vi "add_vi.vi"(8 "error in (no error)":errorcluster, 9 "Path":path, 10 "vi_name":string, 11 "VIGraph in":refnum<class "HierarchyGraph.lvclass">) -> (0 "error out":errorcluster, 1 "VINode out":refnum<class "HierarchyNode.lvclass">, 2 "node already included?":bool, 3 "VIGraph out":refnum<class "HierarchyGraph.lvclass">)   [LabVIEW 2020, in "vi-hierarchy.lvlib" / "HierarchyGraph.lvclass"]
uses:
  HierarchyGraph.lvclass
  C:/Projects/labview-project-load-tools/source/submodules/graph-api-labview/source/api/Graph/Graph.lvclass
  VINode/HierarchyNode.lvclass
  C:/Projects/labview-project-load-tools/source/submodules/graph-api-labview/source/api/Node/Node.lvclass
  HierarchyGraph.lvclass/HierarchyGraph.ctl
  <vilib>/Utility/miscctls.llb/LVMapReplaceAction.ctl
  api/Graph/Graph.lvclass
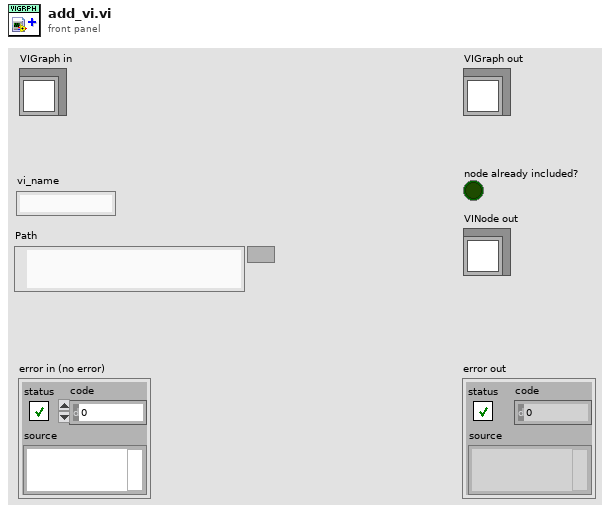
[diagram p1: front panel]
types:
  T1 = typedef "LVMapReplaceAction.ctl" = enum32{"Modify Entry only if found", "Add or Modify Entry", "Delete Entry"}
  T2 = map{string, refnum<class "HierarchyNode.lvclass">}
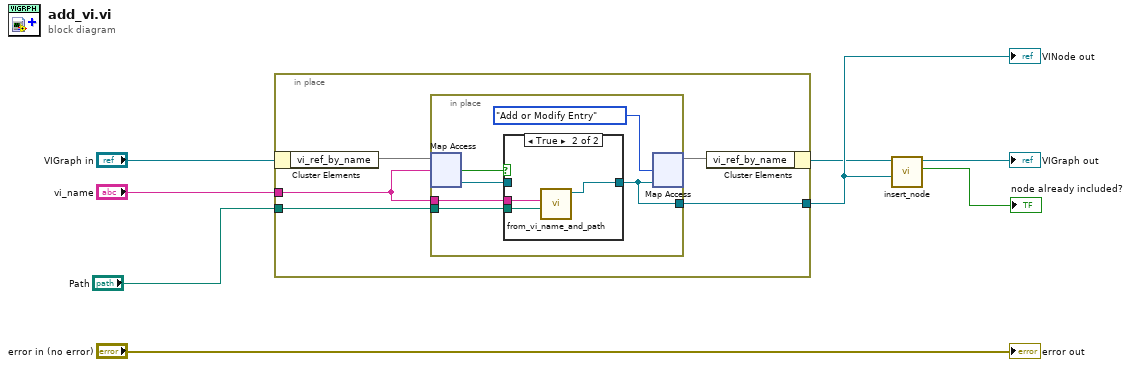
[diagram p0: block diagram]
diagram:
  n1 = in-place {
    in-place-border: "vi_name" -> [w12]
    in-place-border: "Path" -> [w11]
    in-place-border: [w9] -> w3
    n2 = in-place-cluster #1("VIGraph in") -> ("vi_ref_by_name"=w13:T2)
    n3 = in-place {
      in-place-border: w12 -> [w18]
      in-place-border: w11 -> [w17]
      in-place-border: [w15] -> w9
      n4 = in-place-map #2(w13, w12) -> (w16:refnum<class "HierarchyNode.lvclass">, w19:bool)  [unwired: 1 in]
      n5 = case shown="True" w19 {
        tunnel: w18 -> [_ w23]
        tunnel: w17 -> [_ w22]
        tunnel: [w20 w21] -> w15
        tunnel: w16 -> [w20 _]
        frame False {
        }
        frame True {
          n6 = call "from_vi_name_and_path.vi"("vi_path"=w22, "vi_name"=w23) -> ("VINode out"=w21:refnum<class "HierarchyNode.lvclass">)  [unwired: 8 in, 1 out]
        }
      }
      n7 = in-place-map #2(w15, LVMapReplaceAction."Add or Modify Entry" ("action")) -> (w10:T2)  [unwired: 2 out]
    }
    n8 = in-place-cluster #1("vi_ref_by_name"=w10) -> (w1:refnum<class "HierarchyGraph.lvclass">)
  }
  "VINode out" <- w3
  n9 = call "insert_node.vi"("node"=w3, "graph"=w1) -> ("node already included?"=→"node already included?":bool, "graph out"=→"VIGraph out":refnum<class "HierarchyGraph.lvclass">)  [unwired: 7 in, 1 out]
  "error out" <- "error in (no error)"
